vi "SaveFrameToAVI.vi"(10 "IMAQ refnum in":T2, 11 "AVI Refnum in":T1) -> ()   [LabVIEW 2013]
doc: "Adds a timestamp to an image (IMAQ refnum in) and saves it to a video file (AVI refnum in)"
uses:
  <vilib>/vision/Image Controls.llb/IMAQ Image.ctl
  <vilib>/vision/Avi.llb/IMAQ AVI2 Refnum.ctl
  <vilib>/vision/NI_Vision_Development_Module.lvlib
panel:
  # "Adds a timestamp to an image (IMAQ refnum in) and saves it to a video file (AVI refnum in)"
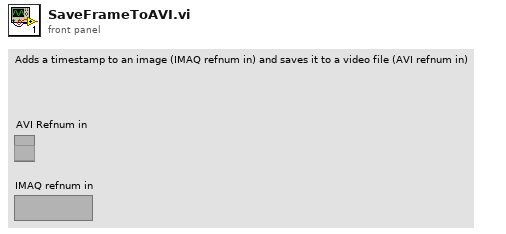
[diagram p1: front panel]
types:
  T1 = typedef "IMAQ AVI2 Refnum.ctl" = refnum<k20>
  T2 = typedef "IMAQ Image.ctl" = refnum<image>
  T3 = cluster{"Desired Font (Application)":enum16{"User-specified Font", "Application Font", "System Font", "Dialog Font"}, "[User-specified Font]":cluster{"Font Name":string, "Size":i16, "Strikeout?":bool, "Italic?":bool, "Underline?":bool, "Outline?":bool, "Shadow?":bool, "Bold?":bool, "Rotation Angle":dbl}, "Horizontal Alignment":i16, "Vertical Alignment":i16}
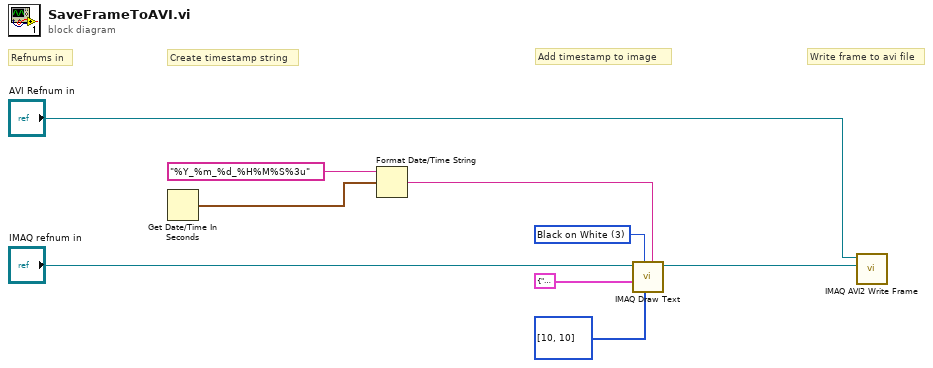
[diagram p0: block diagram]
diagram:
  w5 = 3 items=["White", "Black", "Inverted", "Black on White", "White on Black"] ("Color")
  # "Write frame to avi file"
  # "Add timestamp to image"
  # "Create timestamp string"
  # "Refnums in"
  n1 = Get Date/Time In Seconds() -> (seconds since 1Jan1904=w3:timestamp)
  n2 = Format Date/Time String(time format string (%c)="%Y_%m_%d_%H%M%S%3u", seconds (now)=w3) -> (date/time string=w4:string)  [unwired: 1 in]
  n3 = call "IMAQ Draw Text"("String"=w4, "Insertion Point"=i32[] [10, 10], "Color"=w5, "Font, Size & Style"=T3 {"Desired Font (Application)"=enum."User-specified Font", "[User-specified Font]"={"Font Name"="", "Size"=26, "Strikeout?"=FALSE, "Italic?"=FALSE, "Underline?"=FALSE, "Outline?"=FALSE, "Shadow?"=FALSE, "Bold?"=FALSE, "Rotation Angle"=0.0}, "Horizontal Alignment"=0, "Vertical Alignment"=1}, "Image Src"="IMAQ refnum in") -> ("Image Dst Out"=w2:T2)  [unwired: 3 in, 3 out]
  n4 = call "IMAQ AVI2 Write Frame"("Image"=w2, "AVI Refnum"="AVI Refnum in") -> ()  [unwired: 7 in, 3 out]
